vi "Read Panel Helper.vi"(8 "Error In":errorcluster, 11 "Panel Actor in":refnum<class "Panel Actor.lvclass">) -> (0 "Error Out":errorcluster, 2 "Panel Helper":refnum<class "Panel Helper.lvclass">)   [LabVIEW 2017, in "MGI-Panel Actor.lvlib" / "Panel Actor.lvclass"]
doc: "Reads the Panel Helper for this Panel Actor.\n\nThe Panel Helper is only valid after this actors Pre-Launch init has run. Calling this VI before this will throw an error.\n\n<B>Panel Actor In:</B> Panel Actor object.\n<B>Error In:</B> Describes error conditions that occurred before this VI ran.\n\n<B>Panel Helpert:</B> Panel Helper object.\n<B>Error Out:</B> Contains error information.\n----\nCopyright: MGI 2018\nAuthor: Derek Trepanier"
uses:
  Panel Actor.lvclass
  <vilib>/ErrorRing/Error Ring.xnode
  <vilib>/Utility/error.llb/Error Cluster From Error Code.vi
  panel-manager/Source/Panel Helper/Panel Helper.lvclass
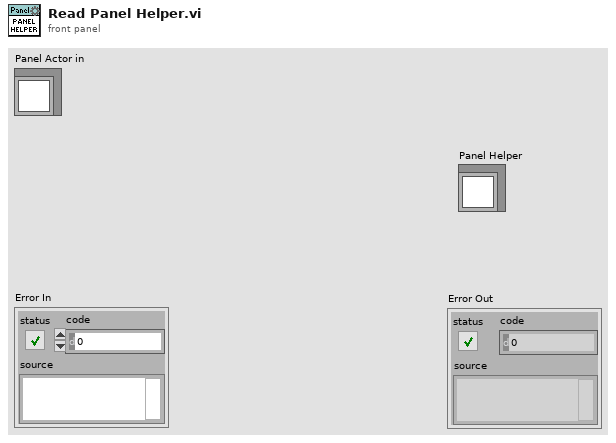
[diagram p1: front panel]
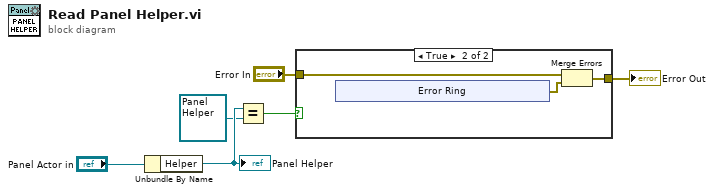
[diagram p0: block diagram]
diagram:
  n1 = Unbundle By Name("Panel Actor in") -> ("Helper"=w5:refnum<class "Panel Helper.lvclass">)
  "Panel Helper" <- w5
  n2 = Equal?(x=w5, y=refnum<class "Panel Helper.lvclass"> refnum) -> (x = y?=w1:bool)
  n3 = case shown="True" w1 {
    tunnel: "Error In" -> [w7 w10]
    tunnel: [w7 w9] -> w2
    frame False {
    }
    frame True {
      n4 = xnode "Error Ring"() -> ("error out"=w8:errorcluster)
      n5 = Merge Errors(w10, w8) -> (w9:errorcluster)
    }
  }
  "Error Out" <- w2
